vi "DepthSense Connect Callback with Input.vi"() -> ()   [LabVIEW 2011]
uses:
  C:/Users/Behavior Room/Desktop/Kinect Mouse/DepthSense/FunctionPointerProxy/FunctionPointerProxy/bin/Release/FunctionPointerProxy.dll
  FunctionPointerProxy/FunctionPointerProxy/bin/Release/FunctionPointerProxy.dll
  <userlib>/libOptrima-2-3/libOptrima-2-3.lvlib
panel:
  out "setting antialiasing worked?":i32(ring)
  out "setting close mode worked?":i32(ring)
  out "setting denoising worked?":i32(ring)
  out "setting leakage worked?":i32(ring)
  out "setting framerate worked?":i32(ring)
  out "error out":errorcluster
  out "camera status":i32(ring)
  out "camera status 2":i32(ring)
  out "framerate":u32
  out "max framerate":u32
  out "min framerate":u32
  out "image height":u32
  out "image width":u32
  out "camera version":string
  in  "User Parameter":variant
  in  "Control Ref":refnum<k24>
  in  "Event Common Data":T1
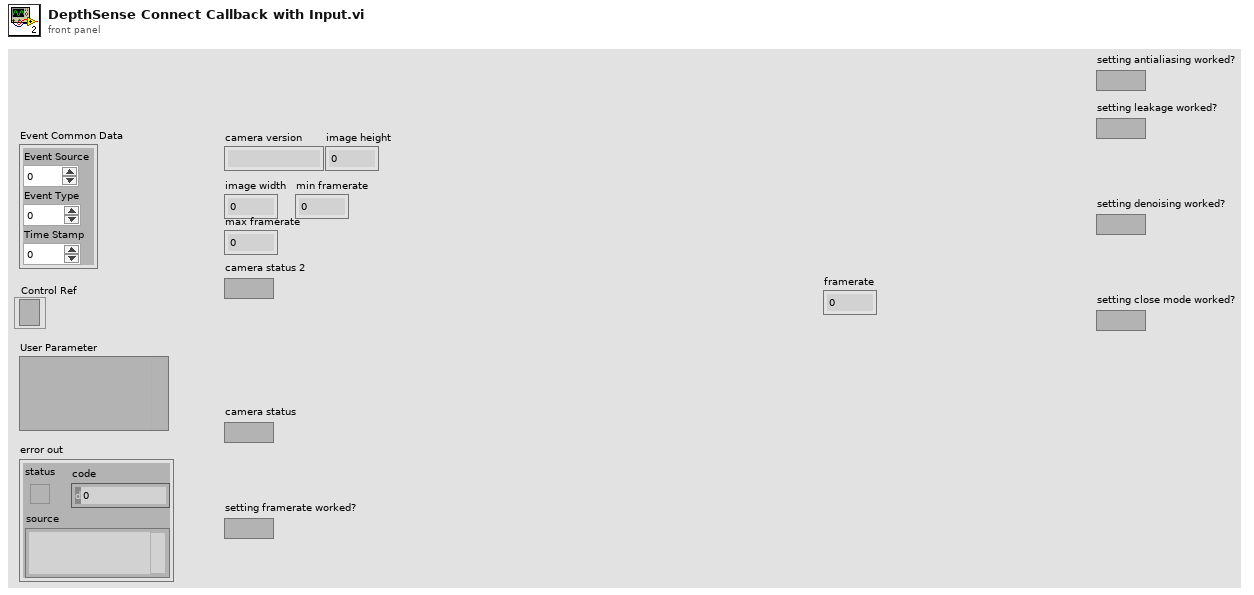
[diagram p1: front panel]
types:
  T1 = cluster{"Event Source":i32, "Event Type":u32, "Time Stamp":u32}
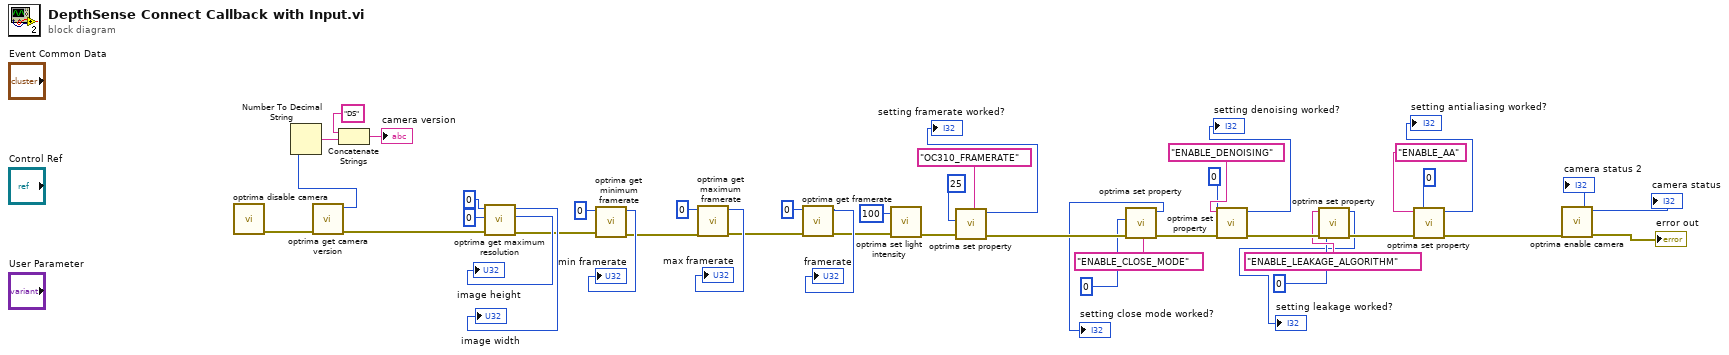
[diagram p0: block diagram]
diagram:
  n1 = call <userlib>:"optrima disable camera.vi"() -> ("error out"=w44:errorcluster)  [unwired: 10 in, 1 out]
  n2 = call <userlib>:"optrima get camera version.vi"("error in (no error)"=w44) -> ("error out"=w18:errorcluster, "version out"=w43:u32)  [unwired: 8 in, 1 out]
  n3 = Number To Decimal String(number=w43) -> (decimal integer string=w42:string)  [unwired: 1 in]
  n4 = Concatenate Strings("DS" ("string"), w42) -> (→"camera version":string)
  n5 = call <userlib>:"optrima get maximum resolution.vi"("error in (no error)"=w18, "rows"=u32 0, "columns"=u32 0) -> ("error out"=w35:errorcluster, "rows out"=→"image height":u32, "columns out"=→"image width":u32)  [unwired: 5 in, 1 out]
  n6 = call <userlib>:"optrima get minimum framerate.vi"("error in (no error)"=w35, "min_framerate"=u32 0) -> ("error out"=w32:errorcluster, "min_framerate out"=→"min framerate":u32)  [unwired: 7 in, 1 out]
  n7 = call <userlib>:"optrima get maximum framerate.vi"("error in (no error)"=w32, "max_framerate"=u32 0) -> ("error out"=w29:errorcluster, "max_framerate out"=→"max framerate":u32)  [unwired: 7 in, 1 out]
  n8 = call <userlib>:"optrima get framerate.vi"("error in (no error)"=w29, "framerate"=u32 0) -> ("error out"=w26:errorcluster, "framerate out"=→"framerate":u32)  [unwired: 7 in, 1 out]
  n9 = call <userlib>:"optrima set light intensity.vi"("error in (no error)"=w26, "intensity_percentage"=u32 100) -> ("error out"=w24:errorcluster)  [unwired: 8 in, 1 out]
  n10 = call <userlib>:"optrima set property.vi"("error in (no error)"=w24, "value"=u32 25, "name"="OC310_FRAMERATE") -> ("error out"=w17:errorcluster, "function return"=→"setting framerate worked?":i32)  [unwired: 7 in]
  n11 = call <userlib>:"optrima set property.vi"("error in (no error)"=w17, "value"=u32 0, "name"="ENABLE_CLOSE_MODE") -> ("error out"=w11:errorcluster, "function return"=→"setting close mode worked?":i32)  [unwired: 7 in]
  n12 = call <userlib>:"optrima set property.vi"("error in (no error)"=w11, "value"=u32 0, "name"="ENABLE_DENOISING") -> ("error out"=w10:errorcluster, "function return"=→"setting denoising worked?":i32)  [unwired: 7 in]
  n13 = call <userlib>:"optrima set property.vi"("error in (no error)"=w10, "value"=u32 0, "name"="ENABLE_LEAKAGE_ALGORITHM") -> ("error out"=w9:errorcluster, "function return"=→"setting leakage worked?":i32)  [unwired: 7 in]
  n14 = call <userlib>:"optrima set property.vi"("error in (no error)"=w9, "value"=u32 0, "name"="ENABLE_AA") -> ("error out"=w16:errorcluster, "function return"=→"setting antialiasing worked?":i32)  [unwired: 7 in]
  n15 = call <userlib>:"optrima enable camera.vi"("error in (no error)"=w16) -> ("error out"=→"error out":errorcluster, "function return"=→"camera status 2" →"camera status":u32)  [unwired: 9 in]
